vi "ReorderBusChannels.vi"(8 "error in (no error)":errorcluster, 11 "Acq Waveforms":waveform(sgl)[](array[waveform])) -> (0 "error out":errorcluster, 2 "Separated Channels":waveform(dbl)[](array[waveform]), 3 "Bus Waveforms":waveform(dbl)[](array[waveform]))   [LabVIEW 2017, in "McsaUtilities.lvlib"]
uses:
  <vilib>/addons/InsightCM/Utilities/MCSA/McsaUtilities.lvlib
  <vilib>/addons/InsightCM/Utilities/Analysis/MCSA/McsaAnalysisFunctions.lvlib
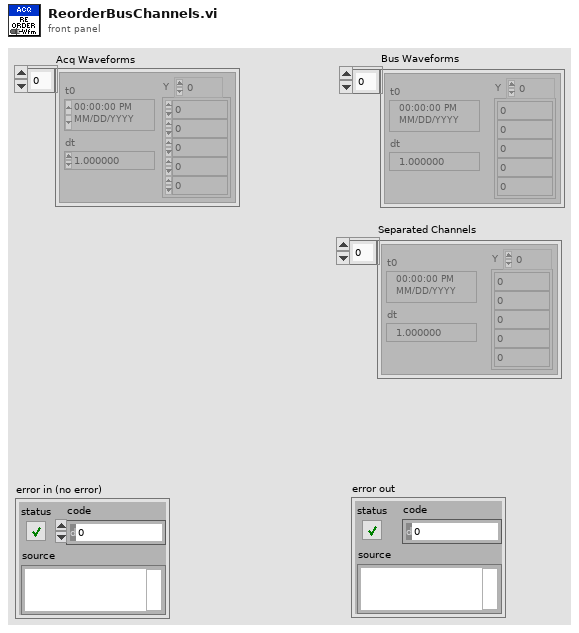
[diagram p1: front panel]
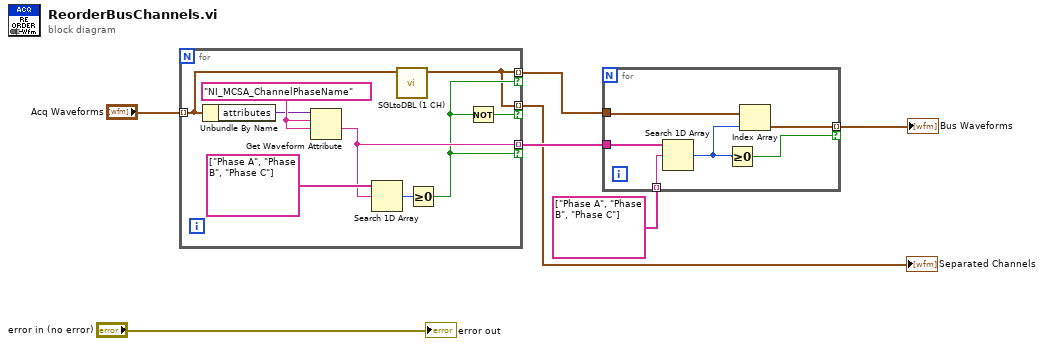
[diagram p0: block diagram]
diagram:
  n1 = for {
    tunnel: "Acq Waveforms" -> [w11] mode=indexing
    tunnel: [w13] -> w6 mode=indexing if=w9
    tunnel: [w8] -> w4 mode=indexing if=w9
    tunnel: [w8] -> w1 mode=indexing if=w10
    w16 = "NI_MCSA_ChannelPhaseName" ("name")
    n2 = Unbundle By Name(w11) -> ("attributes"=w15:variant)
    n3 = Get Waveform Attribute(5:w16, 6:w16, 7:w15) -> (1:w13:string)  [unwired: 1 in, 3 out]
    n4 = Search 1D Array(1D array=string[] ["Phase A", "Phase B", "Phase C"], element=w13) -> (index of element=w12:i32)  [unwired: 1 in]
    n5 = call <vilib>:"SGLtoDBL (1 CH).vi"("Waveform in"=w11) -> ("Waveform out"=w8:waveform(dbl))  [unwired: 10 in]
    n6 = Greater Or Equal To 0?(x=w12) -> (x >= 0?=w9:bool)
    n7 = Not(x=w9) -> (.not. x?=w10:bool)
  }
  "Separated Channels" <- w1
  n8 = for {
    tunnel: w4 -> [w20]
    tunnel: string[] ["Phase A", "Phase B", "Phase C"] -> [w22] mode=indexing
    tunnel: w6 -> [w21]
    tunnel: [w17] -> w2 mode=indexing if=w18
    n9 = Search 1D Array(1D array=w21, element=w22) -> (index of element=w19:i32)  [unwired: 1 in]
    n10 = Greater Or Equal To 0?(x=w19) -> (x >= 0?=w18:bool)
    n11 = Index Array(array=w20, index=w19) -> (element=w17:waveform(dbl))
  }
  "Bus Waveforms" <- w2
  "error out" <- "error in (no error)"
